vi "Subtract.vi"(0 "A":dbl, 5 "B":dbl, 7 "Stop":bool, 11 "Error in":errorcluster) -> (4 "SUB":dbl, 15 "Error out":errorcluster)   [LabVIEW 2020, in "Subpanel access.lvlib"]
uses:
  Subpanel access.lvlib
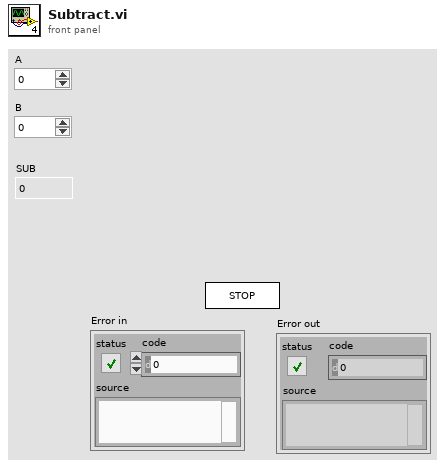
[diagram p1: front panel]
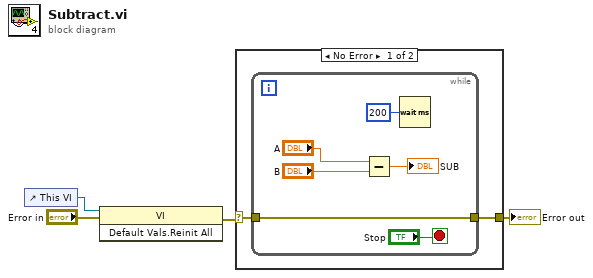
[diagram p0: block diagram]
diagram:
  n1 = control-ref of="This VI"() -> (w1:refnum<vi>)
  n2 = invoke class="VI" method="Default Vals.Reinit All"(reference=w1, error in="Error in") -> (error out=w3:errorcluster)  [unwired: 1 in, 2 out]
  n3 = case shown="No Error" w3 {
    selector: w3 -> [w6 w13]
    tunnel: [w5 w13] -> w4
    frame No Error {
      n4 = while {
        tunnel: [w12] -> w5
        tunnel: w6 -> [w12]
        stop <- "Stop" stop-if-true
        n5 = Subtract(x="A", y="B") -> (x-y=→"SUB":dbl)
        n6 = Wait (ms)(milliseconds to wait=u32 200) -> ()  [unwired: 1 out]
      }
    }
    frame Error {
      # "Do not execute if error"
    }
  }
  "Error out" <- w4
